vi "Report File Close.vi"(8 "error in (no error)":errorcluster, 11 "Report File in":refnum<class "Report File.lvclass">) -> (0 "error out":errorcluster, 3 "Report File out":refnum<class "Report File.lvclass">)   [LabVIEW 2018, in "Report File.lvclass"]
uses:
  Report File.lvclass
  Report File.lvclass/Report File.ctl
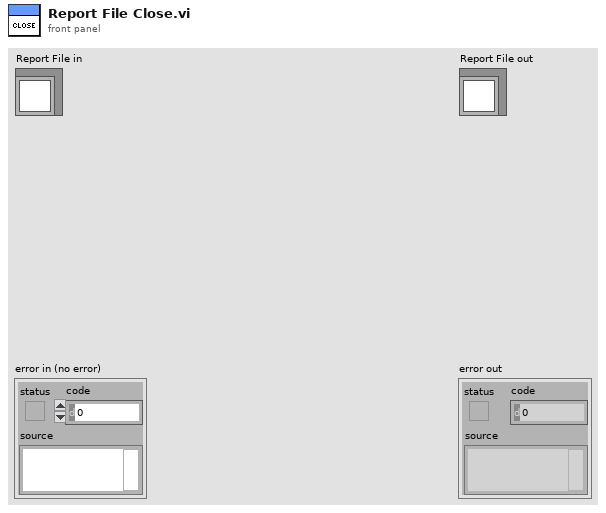
[diagram p1: front panel]
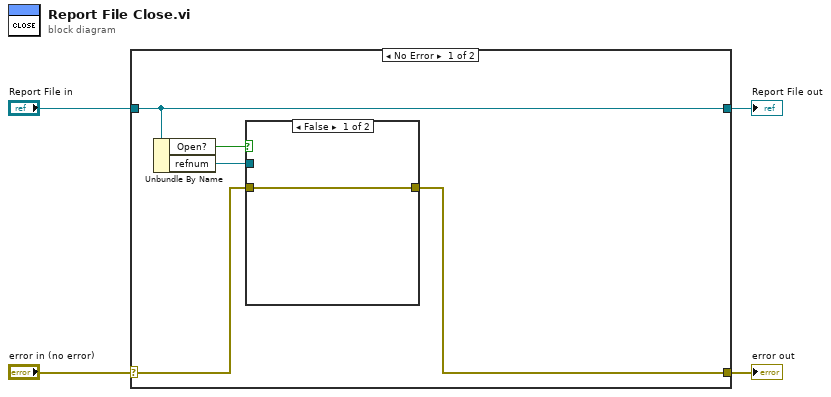
[diagram p0: block diagram]
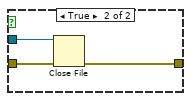
[diagram p2: hidden frame]
diagram:
  n1 = case shown="No Error" "error in (no error)" {
    selector: "error in (no error)" -> [w6 w15]
    tunnel: [w5 w15] -> w3
    tunnel: [w9 w14] -> w1
    tunnel: "Report File in" -> [w9 w14]
    frame No Error {
      n2 = Unbundle By Name(w9) -> ("Open?"=w8:bool, "refnum"=w7:refnum<file>)
      n3 = case shown="False" w8 {
        tunnel: w7 -> [_ w13]
        tunnel: w6 -> [w10 w12]
        tunnel: [w10 w11] -> w5
        frame False {
        }
        frame True {
          n4 = Close File(refnum=w13, error in=w12) -> (error out=w11:errorcluster)  [unwired: 1 out]
        }
      }
    }
    frame Error {
    }
  }
  "error out" <- w3
  "Report File out" <- w1
